vi "test Subset Pointer.vi"(8 "error in (no error)":errorcluster, 11 "TestCase in":refnum<class "Lifecycle Tests.lvclass">) -> (0 "error out":errorcluster, 3 "TestCase out":refnum<class "Lifecycle Tests.lvclass">)   [LabVIEW 2017, in "Pointer Tests.lvlib" / "Lifecycle Tests.lvclass"]
uses:
  Lifecycle Tests.lvclass
  Source/Classes/Pointer/Pointer.lvclass/Pointer.ctl
  Source/Classes/Pointer/Public/New/New (4B).vi
  Source/Classes/Pointer/Public/Write/Write (1D I32).vi
  Source/Classes/Pointer/Public/Read/Read (0D I32).vi
  Source/Classes/Pointer/Public/Write/Write (0D I32).vi
  Source/Classes/Pointer/Private/Allocate.vi
  Source/Classes/Pointer/Protected/Parameter Checking/Check Subset.vi
  Source/Classes/Pointer/API/Accessors/Get Address.vi
  Source/Classes/Pointer/API/Encapsulate External Pointer.vi
  Source/Classes/Pointer/Protected/Parameter Checking/Check Null Pointer.vi
  Source/Classes/Pointer/Public/Write (No Check)/Write (No Check 1D I32).vi
  Source/Classes/Pointer/Protected/Parameter Checking/Check Subset (Power of 2).vi
  Source/Classes/Pointer/Public/Read (No Check)/Read (No Check 0D I32).vi
  Source/Classes/Pointer/Public/Write (No Check)/Write (No Check 0D I32).vi
  Source/Classes/Pointer/Private/Deallocate.vi
  Source/Classes/Pointer/API/Accessors/Set Address.vi
  Source/Classes/Pointer/API/Accessors/Set Size.vi
  Source/Classes/Pointer/Private/Set Internal.vi
  Source/Classes/Pointer/Protected/Errors.vi
  Source/Classes/Pointer/Protected/Error VIs/Out of Bounds.vi
  Source/Classes/Pointer/API/Accessors/Get Size.vi
  Source/Classes/Pointer/Protected/Error VIs/Null Pointer.vi
  Source/Classes/Pointer/Private/Count to Size.vi
  Source/Classes/Pointer/Protected/Get Internal.vi
  Source/Classes/Pointer/Protected/Error VIs/Zone.vi
  Source/VIs/Write String into Source.vi
  Source/Classes/Pointer/Protected/Error Building/Write Pointer Size.vi
  Source/Classes/Pointer/Protected/Error Building/Create Error.vi
  Source/VIs/Write Number into Source.vi
  Source/VIs/VIs for Poly/Write U64 into Source.vi
  Source/Constants/Constants.vi
  Source/Constants/Library Name.vi
  Source/Classes/Pointer/Protected/Error Building/Get Error Info.vi
  Source/VIs/Create Error Cluster.vi
  Source/VIs/VIs for Poly/Create Error Cluster (256B).vi
  Source/VIs/Set Error Status.vi
  Source/VIs/Set Error Code.vi
  Source/VIs/Set Error Source.vi
  Source/Classes/Pointer/Pointer.lvclass
  <vilib>/addons/_JKI Toolkits/VI Tester/TestCase.llb/TestCase.lvclass
  C:/Program Files (x86)/National Instruments/LabVIEW 2017/vi.lib/addons/_JKI Toolkits/VI Tester/TestCase.llb/TestCase.lvclass
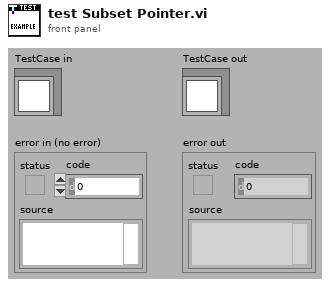
[diagram p1: front panel]
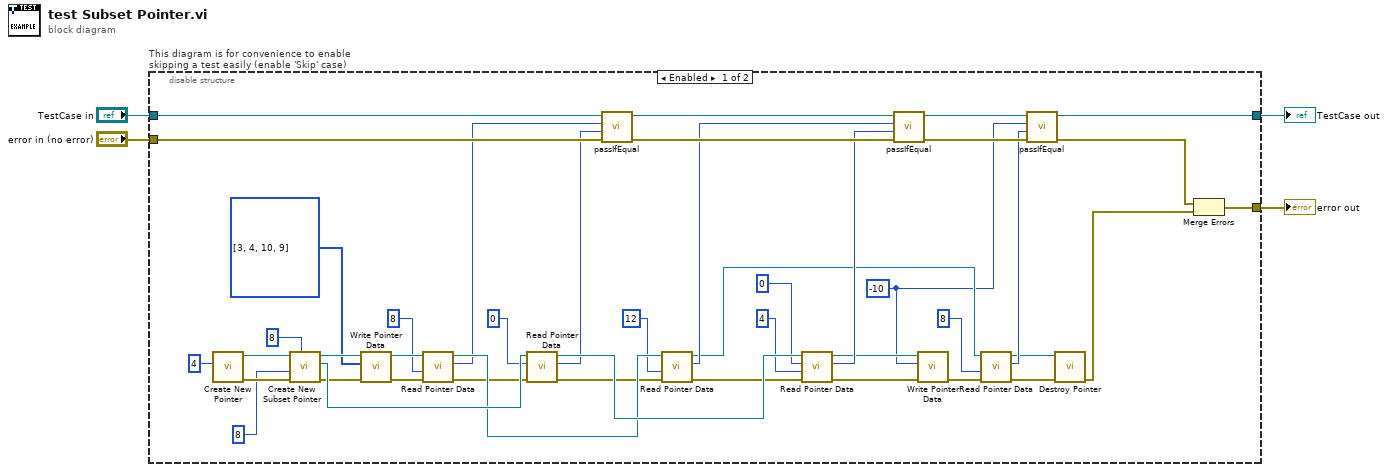
[diagram p0: block diagram]
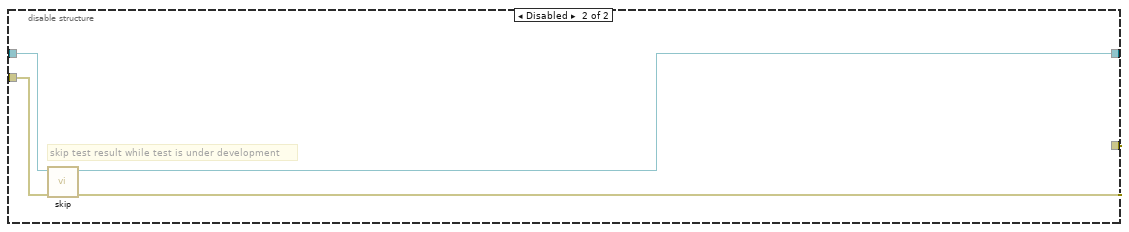
[diagram p2: hidden frame]
diagram:
  n1 = disable-structure "This diagram is for convenience to enable skipping a test easily (enable 'Skip' case)" shown="Enabled" {
    disable-tunnel: "TestCase in" -> [w28 w52]
    disable-tunnel: [w13 w50] -> w1
    disable-tunnel: [w21 w51] -> w3
    disable-tunnel: "error in (no error)" -> [w48 w49]
    frame Enabled {
      w12 = -10 ("length (-1: rest)")
      n2 = call-poly "Create New Pointer.vi"("count (1)"=u64 4) -> ("error out"=w42:errorcluster, "Pointer"=w47:refnum<class "Pointer.lvclass">)  [unwired: 9 in]
      n3 = call "Create New Subset Pointer.vi"("length (-1: rest)"=i64 8, "error in (no error)"=w42, "offset (0)"=u64 8, "base Pointer in"=w47) -> ("error out"=w35:errorcluster, "subset Pointer"=w40:refnum<class "Pointer.lvclass">, "base Pointer out"=w45:refnum<class "Pointer.lvclass">)  [unwired: 4 in, 1 out]
      n4 = call-poly "Write Pointer Data.vi"("error in (no error)"=w35, "buffer in"=i32[] [3, 4, 10, 9] ("length (-1: rest)"), "Pointer in"=w45) -> ("error out"=w41:errorcluster, "Pointer out"=w43:refnum<class "Pointer.lvclass">)  [unwired: 5 in, 2 out]
      n5 = call-poly "Read Pointer Data.vi"("error in (no error)"=w41, "offset (0)"=u64 8, "Pointer in"=w43) -> ("error out"=w9:errorcluster, "value out"=w25:i32, "Pointer out"=w31:refnum<class "Pointer.lvclass">)  [unwired: 5 in, 1 out]
      n6 = call-poly "Read Pointer Data.vi"("error in (no error)"=w9, "value in"=0 ("length (-1: rest)"), "Pointer in"=w40) -> ("error out"=w8:errorcluster, "value out"=w24:i32, "Pointer out"=w34:refnum<class "Pointer.lvclass">)  [unwired: 5 in, 1 out]
      n7 = call-dynamic "passIfEqual.vi"("error in (no error)"=w48, "y"=w24, "x"=w25, "TestCase in"=w28) -> ("error out"=w29:errorcluster, "TestCase out"=w26:refnum<class "Lifecycle Tests.lvclass">)  [unwired: 6 in]
      n8 = call-poly "Read Pointer Data.vi"("error in (no error)"=w8, "offset (0)"=u64 12, "Pointer in"=w31) -> ("error out"=w7:errorcluster, "value out"=w23:i32, "Pointer out"=w16:refnum<class "Pointer.lvclass">)  [unwired: 5 in, 1 out]
      n9 = call-poly "Read Pointer Data.vi"("error in (no error)"=w7, "offset (0)"=u64 4, "value in"=0 ("length (-1: rest)"), "Pointer in"=w34) -> ("error out"=w20:errorcluster, "value out"=w22:i32, "Pointer out"=w18:refnum<class "Pointer.lvclass">)  [unwired: 4 in, 1 out]
      n10 = call-dynamic "passIfEqual.vi"("error in (no error)"=w29, "y"=w22, "x"=w23, "TestCase in"=w26) -> ("error out"=w27:errorcluster, "TestCase out"=w14:refnum<class "Lifecycle Tests.lvclass">)  [unwired: 6 in]
      n11 = call-poly "Write Pointer Data.vi"("error in (no error)"=w20, "value"=w12, "Pointer in"=w18) -> ("error out"=w19:errorcluster)  [unwired: 5 in, 3 out]
      n12 = call-poly "Read Pointer Data.vi"("error in (no error)"=w19, "offset (0)"=u64 8, "Pointer in"=w16) -> ("error out"=w17:errorcluster, "value out"=w10:i32, "Pointer out"=w5:refnum<class "Pointer.lvclass">)  [unwired: 5 in, 1 out]
      n13 = call-dynamic "passIfEqual.vi"("error in (no error)"=w27, "y"=w10, "x"=w12, "TestCase in"=w14) -> ("error out"=w15:errorcluster, "TestCase out"=w13:refnum<class "Lifecycle Tests.lvclass">)  [unwired: 6 in]
      n14 = call "Destroy Pointer.vi"("error in (no error)"=w17, "Pointer in"=w5) -> ("error out"=w6:errorcluster)  [unwired: 8 in, 1 out]
      n15 = Merge Errors(w15, w6) -> (w21:errorcluster)
    }
    frame Disabled {
      # "skip test result while test is under development"
      n16 = call <vilib>:"skip.vi"("error in (no error)"=w49, "TestCase in"=w52) -> ("error out"=w51:errorcluster, "TestCase out"=w50:refnum<class "Lifecycle Tests.lvclass">)  [unwired: 8 in]
    }
  }
  "error out" <- w3
  "TestCase out" <- w1
